vi "Traversal VI Type.vi"(9 "User Data In":variant, 11 "NodeRef":refnum<data-value>) -> (0 "error out":errorcluster, 1 "User Data":variant)   [LabVIEW 2020, in "PicoG-ParserLexer.lvlib"]
uses:
  PicoG-ParserLexer.lvlib
  Node/Node.lvclass
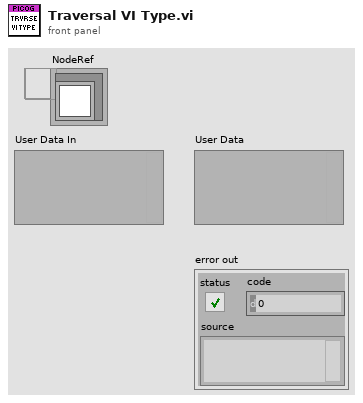
[diagram p1: front panel]
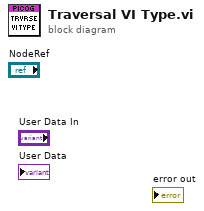
[diagram p0: block diagram]
diagram:
